vi "FPGAmain_5782_Dual_PID_2_channel_3.vi"() -> ()   [LabVIEW 2013]
uses:
  FPGA/DataMode.ctl
  FPGA/Input_5782/5782_states.ctl
  <vilib>/Platform/TimedLoop/XDataNode/timing_clust.ctl
  <vilib>/Platform/TimedLoop/XDataNode/nitl_modes.ctl
  <vilib>/Platform/TimedLoop/XDataNode/wakeup.ctl
  <vilib>/rvi/Emulation/niFpgaSctlEmulationGetInTimedLoop.vi
  <vilib>/rvi/Emulation/niFpgaEmulationReportErrorSimple.vi
  <vilib>/rvi/Emulation/niFpgaGetClockAttributes.vi
  <vilib>/rvi/eio/common/nirviEmuTemplateMethod_errors.vi
  <vilib>/rvi/Emulation/niFpgaCriticalErrorInLSC.vi
  <vilib>/rvi/DataTransferAndStorage/Register/Emulation/niFpgaRegisterEmulationFpgaImpl.vi
  <instcachedir>/0/niFpgaRegisterEmulationFpgaImpl_DCF4BC0110594B98B44A971D60CEEC4D.lvgen/niFpgaRegisterEmulationFpgaImpl_DCF4BC0110594B98B44A971D60CEEC4D_011.vi
  <vilib>/rvi/DataTransferAndStorage/Container/Common/niFpgaContainerGetUniqueNameForEmu.vi
  <instcachedir>/0/niFpgaRegisterEmulationFpgaImpl_DCF4BC0110594B98B44A971D60CEEC4D.lvgen/niFpgaRegisterEmulationFpgaImpl_DCF4BC0110594B98B44A971D60CEEC4D_012.vi
  <instcachedir>/0/niFpgaRegisterEmulationFpgaImpl_DCF4BC0110594B98B44A971D60CEEC4D.lvgen/niFpgaRegisterEmulationFpgaImpl_DCF4BC0110594B98B44A971D60CEEC4D_003.vi
  <instcachedir>/0/niFpgaRegisterEmulationFpgaImpl_DCF4BC0110594B98B44A971D60CEEC4D.lvgen/niFpgaRegisterEmulationFpgaImpl_DCF4BC0110594B98B44A971D60CEEC4D_007.vi
  <instcachedir>/0/niFpgaRegisterEmulationFpgaImpl_DCF4BC0110594B98B44A971D60CEEC4D.lvgen/niFpgaRegisterEmulationFpgaImpl_DCF4BC0110594B98B44A971D60CEEC4D_008.vi
  <instcachedir>/0/niFpgaRegisterEmulationFpgaImpl_DCF4BC0110594B98B44A971D60CEEC4D.lvgen/niFpgaRegisterEmulationFpgaImpl_DCF4BC0110594B98B44A971D60CEEC4D_021.vi
  <instcachedir>/0/niFpgaRegisterEmulationFpgaImpl_DCF4BC0110594B98B44A971D60CEEC4D.lvgen/niFpgaRegisterEmulationFpgaImpl_DCF4BC0110594B98B44A971D60CEEC4D_020.vi
  <instcachedir>/0/niFpgaRegisterEmulationFpgaImpl_DCF4BC0110594B98B44A971D60CEEC4D.lvgen/niFpgaRegisterEmulationFpgaImpl_DCF4BC0110594B98B44A971D60CEEC4D_009.vi
  <vilib>/rvi/FIFO/Fifo_Resource/nirvififoEmulationReadFpgaImpl.vi
  <vilib>/rvi/interface/RandomDataEmulation/nirviRandomDataMultiElementFPGAFIFO.vi
  <instcachedir>/0/nirviRandomDataMultiElementFPGAFIFO_F2B80EDE0D7944A08478D8D26097D4DB.lvgen/nirviRandomDataMultiElementFPGAFIFO_F2B80EDE0D7944A08478D8D26097D4DB_005.vi
  <vilib>/rvi/interface/RandomDataEmulation/niFpgaRandomDataHandleErrors.vi
  <instcachedir>/0/niFpgaRegisterEmulationFpgaImpl_DCF4BC0110594B98B44A971D60CEEC4D.lvgen/niFpgaRegisterEmulationFpgaImpl_DCF4BC0110594B98B44A971D60CEEC4D_013.vi
  <vilib>/rvi/interface/RandomDataEmulation/nirviRandomDataFPGAFIFO.vi
  <vilib>/rvi/FIFO/Fifo_Resource/nirvififoEmulationWriteFpgaImpl.vi
  <vilib>/Platform/TimedLoop/XDataNode/XDataNode.xnode
  <vilib>/eio/EIONode/EIONode.xnode
  <vilib>/rvi/DataTransferAndStorage/Container/XNode/niFpgaContainer.xnode
  <vilib>/rvi/DataTransferAndStorage/Register/Emulation/niFpgaRegisterEmulation.vi
  <vilib>/rvi/FIFO/Fifo_Resource/nirvififoEmulationRead.vi
  <vilib>/rvi/interface/RandomDataEmulation/nirviRandomDataFpgaMultiElementTemplate.vi
  <vilib>/rvi/interface/RandomDataEmulation/nirviRandomDataFpgaReadWriteTemplate.vi
  <vilib>/rvi/FIFO/Fifo_Resource/nirvififoEmulationWrite.vi
  <vilib>/Platform/TimedLoop/XDataNode/XDNodeRunTimeDep.lvlib
panel:
  in  "IO Module\\AO Data Sync":bool=TRUE
  in  "IO Module\\SPI Write Data":u16
  out "IO Module\\SPI Read Data":u8
  in  "IO Module\\SPI Read":bool
  in  "IO Module\\SPI Write":bool
  in  "IO Module\\SPI Address":u16
  in  "IO Module\\SPI Device":u8
  out "IO Module\\SPI Idle":bool
  in  "AM phase":fxp<+,64,64>
  in  "delay phase":fxp<+,64,64>
  in  "User Command Commit":bool
  in  "User Command":u8
  out "User Command Idle":bool
  out "User Command Status":u8
  in  "User Data 0":u8
  in  "User Data 1":u8
  out "PLL Locked":bool
  out "User Error":bool
  out "Configured?":bool
  in  "Continuous":bool
  in  "5782 record length":u16=4000 caption="Samples Per Trigger" min=1 step=1
  in  "Trigger Acquisition":bool
  out "IO Module\\Trigger Input":bool
  in  "Downsample":fxp<+,8,8>=1.0
  in  "new coeffs":bool
  in  "FIR coeffs":fxp<+/-,18,18>[](array[numeric])
  in  "CIC Gain":fxp<+/-,32,1>=0.00390625 format="%#_32g"
  in  "Acquisition running":bool
  in  "Phase output":fxp<+,64,64>[](array[numeric])=[0.0, 0.0, 0.0, 0.0, 0.0, 0.0, 0.0, 0.0]
  in  "Simulated phase 5782":fxp<+,64,64>[](array[numeric])=[0.0, 0.0]
  in  "Mode":T1
  in  "Phase 5782":fxp<+,64,64>[](array[numeric])=[0.0, 0.0]
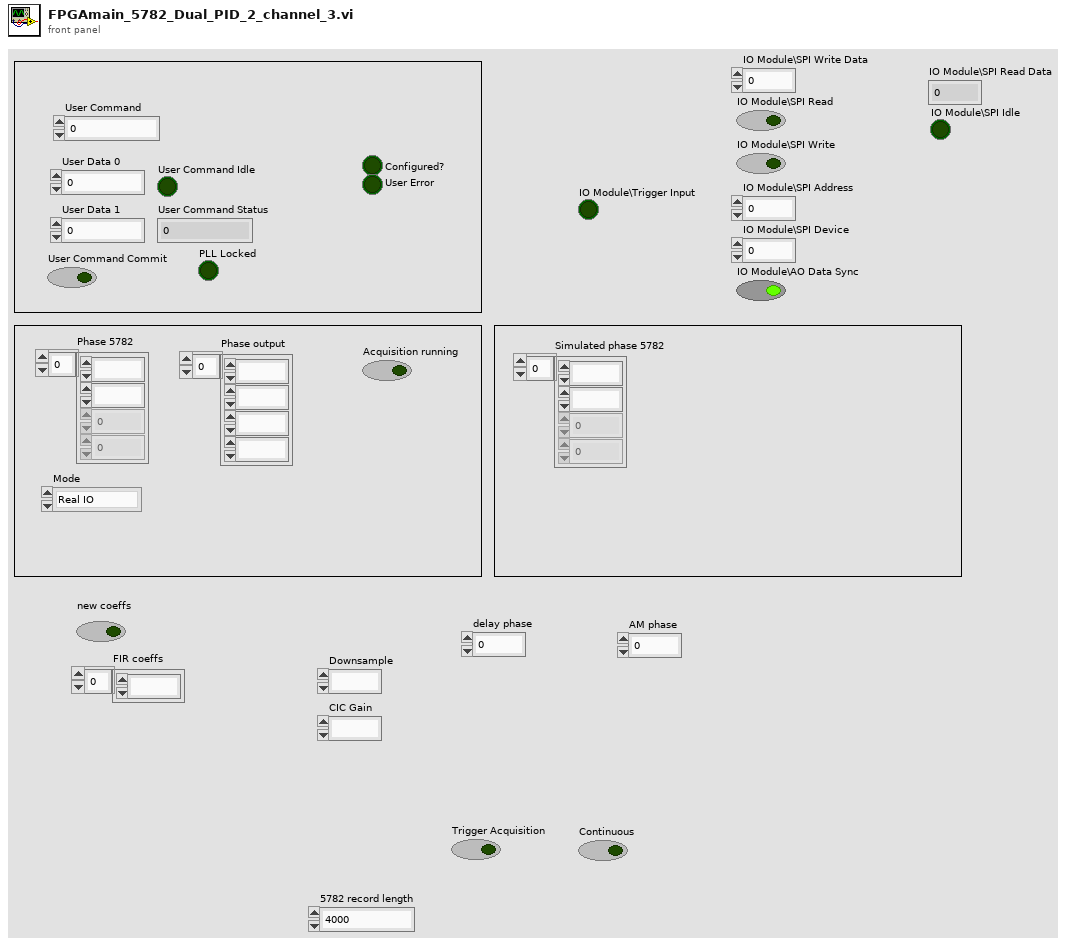
[diagram p1: front panel]
types:
  T1 = typedef "DataMode.ctl" = enum16{"Real IO", "Simulated"}
  T2 = typedef "5782_states.ctl" = enum8{"Wait for trigger", "Acquisition", "Send record length", "Quiet period"}
  T3 = typedef "XDNodeRunTimeDep.lvlib/timing_clust.ctl" = cluster{"Expected End [f-1]":u64, "Actual End [f-1]":u64, "Finished Late? [f-1]":bool, "Expected End [i-1]":u64, "Actual End [i-1]":u64, "Finished Late? [i-1]":bool, "Expected Start [i]":u64, "Actual Start [i]":u64, "Expected Start [f]":u64, "Actual Start [f]":u64, "Source Name":string, "Structure Name":string, "Period":i64, "Deadline":i64, "Offset":i64, "Start":i64, "Priority":i32, "Timeout":i32, "Mode":T4, "Wakeup Reason":T5, "Error":errorcluster, "Source Type":string, "Secondary Source Type":string, "Global End Time":u64, "Global Start Time":u64, "Frame Duration":u64, "Iteration Duration":u64, "Assigned CPU":i32, "I/O Scan Engine Mode":u32}
  T4 = typedef "XDNodeRunTimeDep.lvlib/nitl_modes.ctl" = enum32{"No Change", "Process missed periods, maintain original phase", "Discard missed periods, maintain original phase", "Process missed periods, ignore original phase", "Discard missed periods, ignore original phase"}
  T5 = typedef "XDNodeRunTimeDep.lvlib/wakeup.ctl" = enum32{"Normal", "Aborted", "Asynchronous wakeup", "Timing source error", "Timed loop error", "Timeout"}
  T6 = typedef "I16 array size 2.ctl" = i16[]
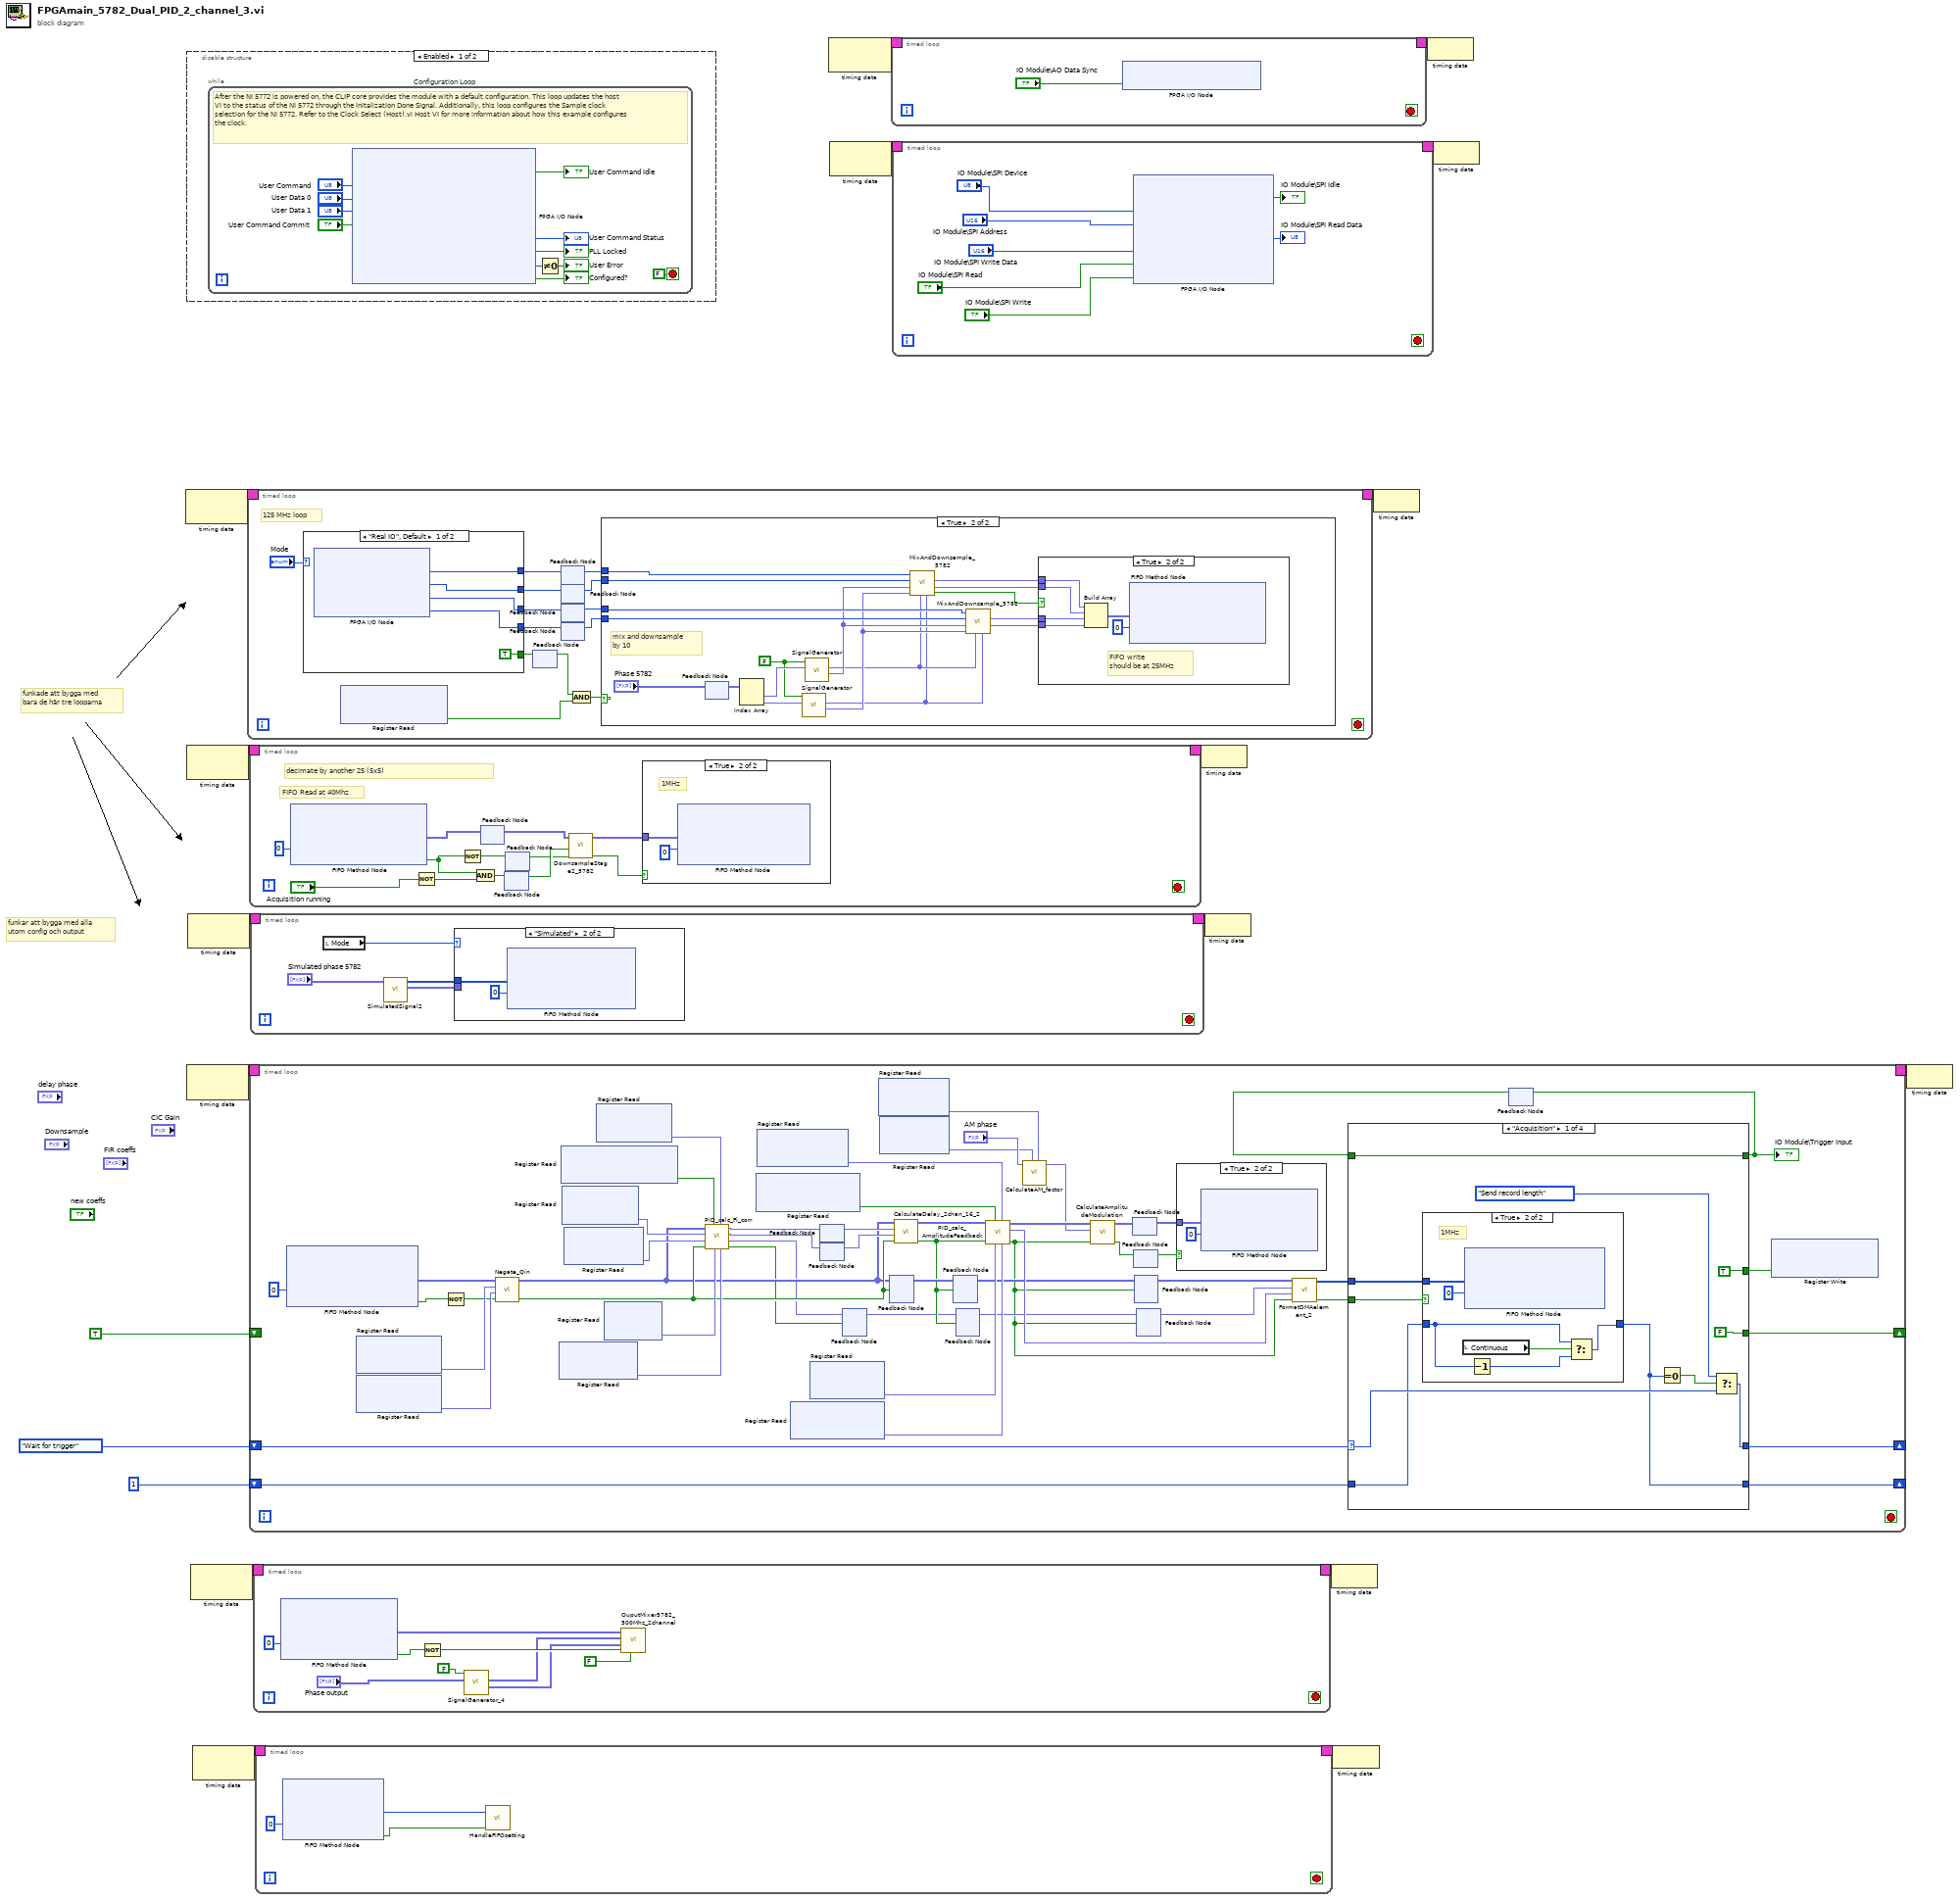
[diagram p0: block diagram]
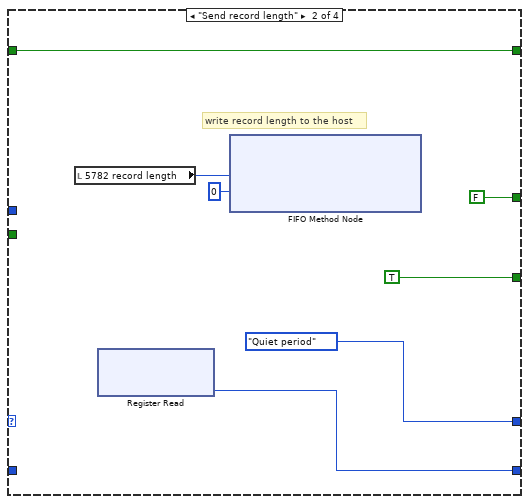
[diagram p4: hidden frame]
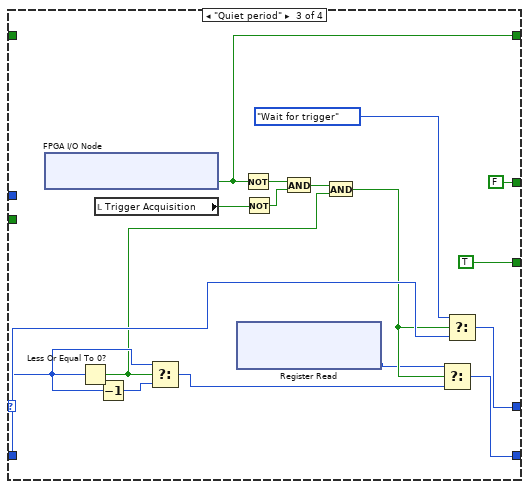
[diagram p5: hidden frame]
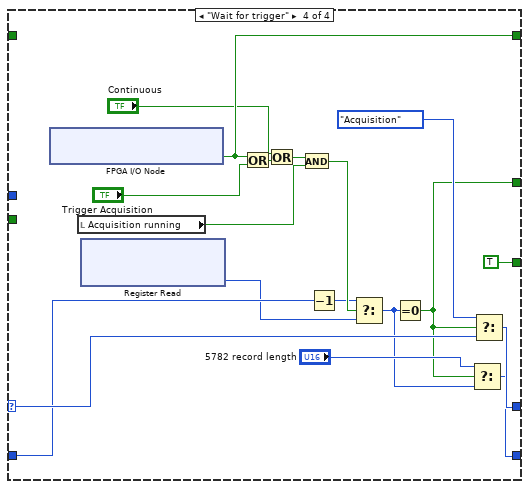
[diagram p6: hidden frame]
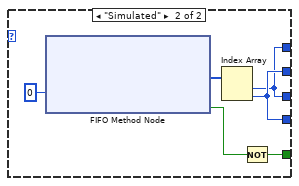
[diagram p10: hidden frame]
diagram:
  # "funkar att bygga med alla\nutom config och output"
  # "funkade att bygga med\nbara de här tre looparna"
  n1 = node-c288() -> (w15:T3)  [unwired: 1 in]
  n2 = disable-structure shown="Enabled" {
    frame Enabled {
      n3 = while "Configuration Loop" {
        stop <- FALSE stop-if-true
        # "After the NI 5772 is powered on, the CLIP core provides the module with a default configuration. This loop updates the host VI to the status of the NI 5772 through the Initalization Done Signal. Additionally, this loop configures the Sample clock selection for the NI 5772. Refer to the Clock Select (Host).vi Host VI for more information about how this example configures the clock."
        n4 = xnode "FPGA I/O Node"("IO Module\\User Command"="User Command", "IO Module\\User Data 0"="User Data 0", "IO Module\\User Data 1"="User Data 1", "IO Module\\User Command Commit"="User Command Commit") -> ("IO Module\\User Command Idle"=→"User Command Idle":bool, "IO Module\\User Command Status"=→"User Command Status":u8, "IO Module\\PLL Locked"=→"PLL Locked":bool, "IO Module\\User Error"=w25:u8, "IO Module\\Initialization Done"=→"Configured?":bool)  [unwired: 9 in, 9 out]
        n5 = Not Equal To 0?(x=w25) -> (x != 0?=→"User Error":bool)
      }
    }
    frame Disabled {
    }
  }
  n6 = node-c288() -> (w19:T3)  [unwired: 1 in]
  n7 = node-c288() -> (w13:T3)  [unwired: 1 in]
  n8 = node-c288() -> (w17:T3)  [unwired: 1 in]
  n9 = node-c288() -> (w6:T3)  [unwired: 1 in]
  n10 = node-c288() -> (w8:T3)  [unwired: 1 in]
  n11 = timed-loop {
    timing: w15 -> [_]
    timing-out: [_] -> w14
    stop <- _ stop-if-true
    # "125 MHz loop"
    n12 = case shown="\"Real IO\", Default" "Mode" {
      tunnel: [w72 w75] -> w41
      tunnel: [w71 w76] -> w39
      tunnel: [w70 w75] -> w37
      tunnel: [w69 w76] -> w34
      tunnel: [TRUE w73] -> w33
      frame "Real IO", Default {
        n13 = xnode "FPGA I/O Node"() -> ("IO Module\\AI 0 N-1"=w72:i16, "IO Module\\AI 0 N"=w71:i16, "IO Module\\AI 1 N-1"=w70:i16, "IO Module\\AI 1 N"=w69:i16)  [unwired: 4 in, 4 out]
      }
      frame "Simulated" {
        n14 = xnode ("FIFO Method Node")("Timeout"=0) -> ("Element"=w77:i16[], "Timed Out?"=w74:bool)  [unwired: 1 in, 1 out]
        n15 = Index Array(array=w77) -> (element #1=w75:i16, element #2=w76:i16)  [unwired: 2 in]
        n16 = Not(x=w74) -> (.not. x?=w73:bool)
      }
    }
    n17 = xnode ("Register Read")() -> ("Data"=w31:bool)  [unwired: 1 in, 1 out]
    n18 = feedback #1() -> (w32:bool)  [unwired: 1 in]
    n19 = feedback-in #1(w33) -> ()
    n20 = feedback #2() -> (w40:i16)  [unwired: 1 in]
    n21 = feedback-in #2(w41) -> ()
    n22 = feedback #3() -> (w38:i16)  [unwired: 1 in]
    n23 = feedback-in #3(w39) -> ()
    n24 = feedback #4() -> (w36:i16)  [unwired: 1 in]
    n25 = feedback-in #4(w37) -> ()
    n26 = feedback #5() -> (w35:i16)  [unwired: 1 in]
    n27 = feedback-in #5(w34) -> ()
    n28 = And(x=w32, y=w31) -> (x .and. y?=w42:bool)
    n29 = case shown="True" w42 {
      tunnel: w40 -> [_ w51]
      tunnel: w38 -> [_ w50]
      tunnel: w36 -> [_ w49]
      tunnel: w35 -> [_ w48]
      frame False {
      }
      frame True {
        w52 = FALSE
        # "mix and downsample\nby 10"
        n30 = feedback #6() -> (w55:fxp<+,64,64>[])  [unwired: 1 in]
        n31 = feedback-in #6("Phase 5782") -> ()
        n32 = Index Array(array=w55) -> (element #1=w54:fxp<+,64,64>, element #2=w56:fxp<+,64,64>)  [unwired: 2 in]
        n33 = call "SignalGenerator.vi"("phase"=w56, "Reset"=w52) -> ("Cos"=w46:fxp<+/-,16,0>, "Sin"=w44:fxp<+/-,16,0>)  [unwired: 7 in, 1 out]
        n34 = call "SignalGenerator.vi"("phase"=w54, "Reset"=w52) -> ("Cos"=w47:fxp<+/-,16,0>, "Sin"=w45:fxp<+/-,16,0>)  [unwired: 7 in, 1 out]
        n35 = call "MixAndDownsample_5782.vi"("sin1"=w44, "sin0"=w45, "cos1"=w46, "cos0"=w47, "signal 1"=w50, "signal 0"=w51) -> ("data valid"=w59:bool, "Q out"=w60:fxp<+/-,16,14>, "I out"=w61:fxp<+/-,16,14>)  [unwired: 3 in]
        n36 = call "MixAndDownsample_5782.vi"("sin1"=w44, "sin0"=w45, "cos1"=w46, "cos0"=w47, "signal 1"=w48, "signal 0"=w49) -> ("Q out"=w57:fxp<+/-,16,14>, "I out"=w58:fxp<+/-,16,14>)  [unwired: 3 in, 1 out]
        n37 = case shown="True" w59 {
          tunnel: w60 -> [_ w67]
          tunnel: w61 -> [_ w64]
          tunnel: w58 -> [_ w63]
          tunnel: w57 -> [_ w62]
          frame False {
          }
          frame True {
            # "FIFO write\nshould be at 25MHz"
            n38 = Build Array(w64, w67, w63, w62) -> (w66:fxp<+/-,16,14>[])
            n39 = xnode ("FIFO Method Node")("Element"=w66, "Timeout"=0) -> ()  [unwired: 1 in, 2 out]
          }
        }
      }
    }
  }
  n40 = timed-loop {
    timing: w19 -> [_]
    timing-out: [_] -> w18
    stop <- _ stop-if-true
    # "FIFO Read at 40Mhz"
    # "decimate by another 25 (5x5)"
    n41 = xnode ("FIFO Method Node")("Timeout"=0) -> ("Element"=w86:fxp<+/-,16,14>[], "Timed Out?"=w88:bool)  [unwired: 1 in, 1 out]
    n42 = Not(x="Acquisition running") -> (.not. x?=w89:bool)
    n43 = Not(x=w88) -> (.not. x?=w82:bool)
    n44 = And(x=w88, y=w89) -> (x .and. y?=w84:bool)
    n45 = feedback #7() -> (w85:fxp<+/-,16,14>[])  [unwired: 1 in]
    n46 = feedback-in #7(w86) -> ()
    n47 = feedback #8() -> (w83:bool)  [unwired: 1 in]
    n48 = feedback-in #8(w84) -> ()
    n49 = feedback #9() -> (w81:bool)  [unwired: 1 in]
    n50 = feedback-in #9(w82) -> ()
    n51 = call "DownsampleStage2_5782.vi"("valid in"=w81, "reset"=w83, "Data in"=w85) -> ("valid out"=w90:bool, "data out"=w91:fxp<+/-,16,14>[])  [unwired: 7 in]
    n52 = case shown="True" w90 {
      tunnel: w91 -> [_ w93]
      frame False {
      }
      frame True {
        # "1MHz"
        n53 = xnode ("FIFO Method Node")("Element"=w93, "Timeout"=0) -> ()  [unwired: 1 in, 2 out]
      }
    }
  }
  n54 = timed-loop {
    timing: w13 -> [_]
    timing-out: [_] -> w12
    shift-right: [w147] -> _
    shift-left: 5782_states."Wait for trigger" ("5782 states") -> [w149]
    shift-right: [w146] -> _
    shift-left: u16 1 ("trigger samples") -> [w148]
    shift-right: [w141] -> _
    shift-left: TRUE -> [_]
    stop <- _ stop-if-true
    n55 = xnode ("FIFO Method Node")("Timeout"=0) -> ("Element"=w127:fxp<+/-,16,14>[], "Timed Out?"=w144:bool)  [unwired: 1 in, 1 out]
    n56 = xnode ("Register Read")() -> ("Data"=w134:fxp<+/-,16,14>)  [unwired: 1 in, 1 out]
    n57 = xnode ("Register Read")() -> ("Data"=w135:fxp<+/-,16,14>)  [unwired: 1 in, 1 out]
    n58 = Not(x=w144) -> (.not. x?=w128:bool)
    n59 = call "Negate_Qin.vi"("valid in"=w128, "DC offset chan 1"=w134, "DC offset chan 0"=w135, "Data in"=w127) -> ("valid out"=w114:bool, "Data out"=w113:fxp<+/-,16,14>[])  [unwired: 6 in]
    n60 = xnode ("Register Read")() -> ("Data"=w121:fxp<+/-,32,4>)  [unwired: 1 in, 1 out]
    n61 = xnode ("Register Read")() -> ("Data"=w118:bool)  [unwired: 1 in, 1 out]
    n62 = xnode ("Register Read")() -> ("Data"=w119:fxp<+/-,32,4>)  [unwired: 1 in, 1 out]
    n63 = xnode ("Register Read")() -> ("Data"=w120:fxp<+/-,32,4>)  [unwired: 1 in, 1 out]
    n64 = xnode ("Register Read")() -> ("Data"=w117:fxp<+/-,32,4>)  [unwired: 1 in, 1 out]
    n65 = xnode ("Register Read")() -> ("Data"=w122:fxp<+/-,32,4>)  [unwired: 1 in, 1 out]
    n66 = call "PID_calc_Fi_corr.vi"("Kd/Tau"=w121, "Ki*Tau"=w117, "Kp"=w122, "Enabled"=w118, "input valid"=w114, "Fi_delta"=w120, "Fi_start"=w119, "Data in"=w113) -> ("output valid"=w111:bool, "c out"=w112:fxp<+/-,32,4>, "cos_fi_korr"=w115:fxp<+/-,16,2>, "sin fi_korr"=w116:fxp<+/-,16,2>)
    n67 = xnode ("Register Read")() -> ("Data"=w132:bool)  [unwired: 1 in, 1 out]
    n68 = xnode ("Register Read")() -> ("Data"=w129:fxp<+/-,32,6>)  [unwired: 1 in, 1 out]
    n69 = xnode ("Register Read")() -> ("Data"=w130:fxp<+/-,32,6>)  [unwired: 1 in, 1 out]
    n70 = xnode ("Register Read")() -> ("Data"=w131:fxp<+/-,32,6>)  [unwired: 1 in, 1 out]
    n71 = feedback-in #10(w116) -> ()
    n72 = feedback #10() -> (w137:fxp<+/-,16,2>)  [unwired: 1 in]
    n73 = feedback #11() -> (w136:fxp<+/-,16,2>)  [unwired: 1 in]
    n74 = feedback-in #11(w115) -> ()
    n75 = feedback #12() -> (w106:fxp<+/-,32,4>)  [unwired: 1 in]
    n76 = feedback-in #12(w112, w111) -> ()
    n77 = xnode ("Register Read")() -> ("Data"=w99:fxp<+/-,16,2>)  [unwired: 1 in, 1 out]
    n78 = xnode ("Register Read")() -> ("Data"=w100:fxp<+/-,16,2>)  [unwired: 1 in, 1 out]
    n79 = feedback #13() -> (w109:fxp<+/-,16,14>[])  [unwired: 1 in]
    n80 = feedback-in #13(w113, w114) -> ()
    n81 = call "CalculateDelay_2chan_16_2.vi"("input valid"=w114, "cos_fi"=w136, "sin fi"=w137, "Data in"=w113) -> ("output valid"=w107:bool, "Data out"=w133:fxp<+/-,16,14>[])  [unwired: 6 in]
    n82 = feedback #14() -> (w108:fxp<+/-,16,14>[])  [unwired: 1 in]
    n83 = feedback-in #14(w109, w107) -> ()
    n84 = feedback #15() -> (w105:fxp<+/-,32,4>)  [unwired: 1 in]
    n85 = feedback-in #15(w106, w107) -> ()
    n86 = call "PID_calc_AmplitudeFeedback.vi"("Kd/Tau"=w130, "Ki*Tau"=w129, "Kp"=w131, "Enabled"=w132, "input valid"=w107, "Data in"=w133) -> ("output valid"=w102:bool, "c(t)"=w123:fxp<+/-,32,21>, "data out"=w104:fxp<+/-,16,14>[])  [unwired: 2 in, 1 out]
    n87 = call "CalculateAM_factor.vi"("b_am"=w99, "a_am"=w100, "AM phase"="AM phase") -> ("AM_factor"=w98:fxp<+/-,16,2>)  [unwired: 7 in, 1 out]
    n88 = call "CalculateAmplitudeModulation.vi"("input valid"=w102, "AM_factor"=w98, "Data in"=w104) -> ("output valid"=w97:bool, "Data out"=w103:fxp<+/-,16,14>[])  [unwired: 7 in]
    n89 = feedback #16() -> (w126:fxp<+/-,16,14>[])  [unwired: 1 in]
    n90 = feedback-in #16(w103) -> ()
    n91 = feedback #17() -> (w125:bool)  [unwired: 1 in]
    n92 = feedback-in #17(w97) -> ()
    n93 = feedback #18() -> (w124:fxp<+/-,16,14>[])  [unwired: 1 in]
    n94 = feedback-in #18(w108, w102) -> ()
    n95 = feedback #19() -> (w110:fxp<+/-,32,4>)  [unwired: 1 in]
    n96 = feedback-in #19(w105, w102) -> ()
    n97 = case shown="True" w125 {
      tunnel: w126 -> [_ w150]
      frame False {
      }
      frame True {
        n98 = xnode ("FIFO Method Node")("Element"=w150, "Timeout"=0) -> ()  [unwired: 1 in, 2 out]
      }
    }
    n99 = call "FormatDMAelement_2.vi"("valid in"=w102, "c(t) - AM"=w123, "c(t) - Phase"=w110, "Data in"=w124) -> ("valid out"=w142:bool, "Element"=w143:u64[])  [unwired: 6 in]
    n100 = feedback #20() -> (w139:bool)  [unwired: 1 in]
    n101 = case shown="\"Acquisition\"" w149 {
      selector: w149 -> [w162 _ w192 w211]
      tunnel: w148 -> [w158 _ w180 w198]
      tunnel: [w161 5782_states."Quiet period" ("5782 states") w191 w210] -> w147
      tunnel: [w155 w170 w193 w209] -> w146
      tunnel: w143 -> [w156 _ _ _]
      tunnel: w142 -> [w157 _ _ _]
      tunnel: [FALSE TRUE TRUE TRUE] -> w141
      tunnel: [TRUE FALSE ("5782 triggered") FALSE ("5782 triggered") w202] -> w140
      tunnel: [w154 w171 w182 w201] -> w138
      tunnel: w139 -> [w154 w171 _ _]
      frame "Acquisition" {
        n102 = case shown="True" w157 {
          tunnel: w156 -> [_ w169]
          tunnel: [w163 w166] -> w155
          tunnel: w158 -> [w163 w164]
          frame False {
          }
          frame True {
            # "1MHz"
            n103 = local read "Continuous"() -> (w167:bool)
            n104 = xnode ("FIFO Method Node")("Element"=w169, "Timeout"=0) -> ()  [unwired: 1 in, 2 out]
            n105 = Decrement(x=w164) -> (x-1=w165:u16)
            n106 = Select(t=w164, s=w167, f=w165) -> (s? t:f=w166:u16)
          }
        }
        n107 = Equal To 0?(x=w155) -> (x = 0?=w159:bool)
        n108 = Select(t=5782_states."Send record length" ("5782 states"), s=w159, f=w162) -> (s? t:f=w161:T2)
      }
      frame "Send record length" {
        # "write record length to the host"
        n109 = local read "5782 record length"() -> (w173:u16)
        n110 = xnode ("Register Read")() -> ("Data"=w170:u16)  [unwired: 1 in, 1 out]
        n111 = xnode ("FIFO Method Node")("Element"=w173, "Timeout"=0) -> ()  [unwired: 1 in, 2 out]
      }
      frame "Quiet period" {
        n112 = xnode "FPGA I/O Node"() -> ("IO Module\\Trigger Input"=w182:bool)  [unwired: 1 in, 1 out]
        n113 = Less Or Equal To 0?(x=w180) -> (x <= 0?=w179:bool)
        n114 = local read "Trigger Acquisition"() -> (w188:bool)
        n115 = Decrement(x=w180) -> (x-1=w181:u16)
        n116 = Select(t=w180, s=w179, f=w181) -> (s? t:f=w178:u16)
        n117 = xnode ("Register Read")() -> ("Data"=w177:u16)  [unwired: 1 in, 1 out]
        n118 = Not(x=w182) -> (.not. x?=w187:bool)
        n119 = Not(x=w188) -> (.not. x?=w186:bool)
        n120 = And(x=w187, y=w186) -> (x .and. y?=w185:bool)
        n121 = And(x=w185, y=w179) -> (x .and. y?=w190:bool)
        n122 = Select(t=w177, s=w190, f=w178) -> (s? t:f=w193:u16)
        n123 = Select(t=5782_states."Wait for trigger" ("5782 states"), s=w190, f=w192) -> (s? t:f=w191:T2)
      }
      frame "Wait for trigger" {
        n124 = xnode "FPGA I/O Node"() -> ("IO Module\\Trigger Input"=w201:bool)  [unwired: 1 in, 1 out]
        n125 = local read "Acquisition running"() -> (w203:bool)
        n126 = xnode ("Register Read")() -> ("Data"=w194:u16)  [unwired: 1 in, 1 out]
        n127 = Or(x=w201, y="Trigger Acquisition") -> (x .or. y?=w197:bool)
        n128 = Or(x="Continuous", y=w197) -> (x .or. y?=w195:bool)
        n129 = And(x=w195, y=w203) -> (x .and. y?=w204:bool)
        n130 = Decrement(x=w198) -> (x-1=w199:u16)
        n131 = Select(t=w199, s=w204, f=w194) -> (s? t:f=w200:u16)
        n132 = Equal To 0?(x=w200) -> (x = 0?=w202:bool)
        n133 = Select(t="5782 record length", s=w202, f=w200) -> (s? t:f=w209:u16)
        n134 = Select(t=5782_states."Acquisition" ("5782 states"), s=w202, f=w211) -> (s? t:f=w210:T2)
      }
    }
    "IO Module\\Trigger Input" <- w138
    n135 = feedback-in #20(w138) -> ()
    n136 = xnode ("Register Write")("Data"=w140) -> ()  [unwired: 1 in, 1 out]
  }
  n137 = timed-loop {
    timing: w17 -> [_]
    timing-out: [_] -> w16
    stop <- _ stop-if-true
    n138 = local read "Mode"() -> (w217:T1)
    n139 = call "SimulatedSignal2.vi"("Phase"="Simulated phase 5782") -> ("dummy do not use"=w214:fxp<+/-,16,0>[], "output"=w216:T6)  [unwired: 9 in]
    n140 = case shown="\"Simulated\"" w217 {
      tunnel: w216 -> [_ w218]
      tunnel: w214 -> [_ _]
      frame "Real IO", Default {
      }
      frame "Simulated" {
        n141 = xnode ("FIFO Method Node")("Element"=w218, "Timeout"=0) -> ()  [unwired: 1 in, 2 out]
      }
    }
  }
  n142 = timed-loop {
    timing: w6 -> [_]
    timing-out: [_] -> w5
    stop <- _ stop-if-true
    n143 = xnode ("FIFO Method Node")("Timeout"=0) -> ("Element"=w226:fxp<+/-,16,14>[], "Timed Out?"=w229:bool)  [unwired: 1 in, 1 out]
    n144 = Not(x=w229) -> (.not. x?=w225:bool)
    n145 = call "SignalGenerator_4.vi"("Phase"="Phase output", "reset"=FALSE) -> ("Sine out"=w222:fxp<+/-,16,0>[], "Cosine out"=w223:fxp<+/-,16,0>[])  [unwired: 8 in]
    n146 = call "OuputMixer5782_500Mhz_2channel.vi"("reset"=FALSE, "valid in"=w225, "Sine in"=w222, "Cosine in"=w223, "Data in"=w226) -> ()  [unwired: 6 in, 1 out]
  }
  n147 = timed-loop {
    timing: w8 -> [_]
    timing-out: [_] -> w7
    stop <- _ stop-if-true
    n148 = xnode ("FIFO Method Node")("Timeout"=0) -> ("Element"=w234:u64, "Timed Out?"=w233:bool)  [unwired: 1 in, 1 out]
    n149 = call "HandleFIFOsetting.vi"("timed out"=w233, "Value"=w234) -> ()  [unwired: 10 in]
  }
  n150 = node-c288() -> (w2:T3)  [unwired: 1 in]
  n151 = node-c288() -> (w4:T3)  [unwired: 1 in]
  n152 = timed-loop {
    timing: w2 -> [_]
    timing-out: [_] -> w1
    stop <- _ stop-if-true
    n153 = xnode "FPGA I/O Node"("IO Module\\AO Data Sync"="IO Module\\AO Data Sync") -> ()  [unwired: 1 in, 1 out]
  }
  n154 = timed-loop {
    timing: w4 -> [_]
    timing-out: [_] -> w3
    stop <- _ stop-if-true
    n155 = xnode "FPGA I/O Node"("IO Module\\SPI Device"="IO Module\\SPI Device", "IO Module\\SPI Address"="IO Module\\SPI Address", "IO Module\\SPI Write Data"="IO Module\\SPI Write Data", "IO Module\\SPI Read"="IO Module\\SPI Read", "IO Module\\SPI Write"="IO Module\\SPI Write") -> ("IO Module\\SPI Idle"=→"IO Module\\SPI Idle":bool, "IO Module\\SPI Read Data"=→"IO Module\\SPI Read Data":u8)  [unwired: 7 in, 7 out]
  }
  n156 = node-c288(w18) -> ()
  n157 = node-c288(w16) -> ()
  n158 = node-c288(w5) -> ()
  n159 = node-c288(w7) -> ()
  n160 = node-c288(w14) -> ()
  n161 = node-c288(w1) -> ()
  n162 = node-c288(w3) -> ()
  n163 = node-c288(w12) -> ()
